vi "Logic.vi"(8 "error in (no error)":errorcluster, 11 "CIFTemplatePlugin in":refnum<class "TemplatePlugin.lvclass">) -> (0 "error out":errorcluster, 3 "CIFTemplatePlugin out":refnum<class "TemplatePlugin.lvclass">)   [LabVIEW 2021, in "TemplatePlugin.lvclass"]
uses:
  TemplatePlugin.lvclass
  D:/dev/CIF-LVCore/src/CIFCore/Class/CIFCorePlugin.lvclass
  TemplatePlugin.lvclass/TemplatePlugin.ctl
  Common/Typedef/Channels.ctl
  CIF-LVCore/src/CIFCore/Class/CIFCorePlugin.lvclass/CIFCorePlugin.ctl
  CIF-LVCore/src/CIFCore/Class/Accessors/Monitor/Write Double 1.vi
  CIF-LVCore/src/CIFCore/Class/Accessors/Monitor/Write U64 1.vi
  CIF-LVCore/src/CIFCore/Class/Accessors/Monitor/Write U64 2.vi
  CIF-LVCore/src/CIFCore/Class/Accessors/Monitor/Write I64 1.vi
  CIF-LVCore/src/CIFCore/Class/Accessors/Monitor/Write I64 2.vi
  <vilib>/CIF Foundation/CIF Channels Core/CIFChannels/CIFChannels.lvclass
  CIF-LVCore/src/CIFCore/Class/CIFCorePlugin.lvclass
  Common/TemplateCommon.lvlib
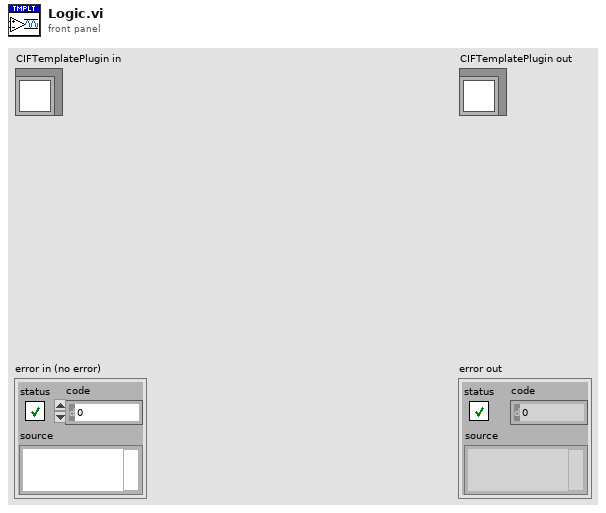
[diagram p1: front panel]
types:
  T1 = typedef "TemplateCommon.lvlib/Channels.ctl" = enum16{"doubleout", "doublein1", "doublein2", "uint_out", "uint_in", "u8array_out", "u8array_in"}
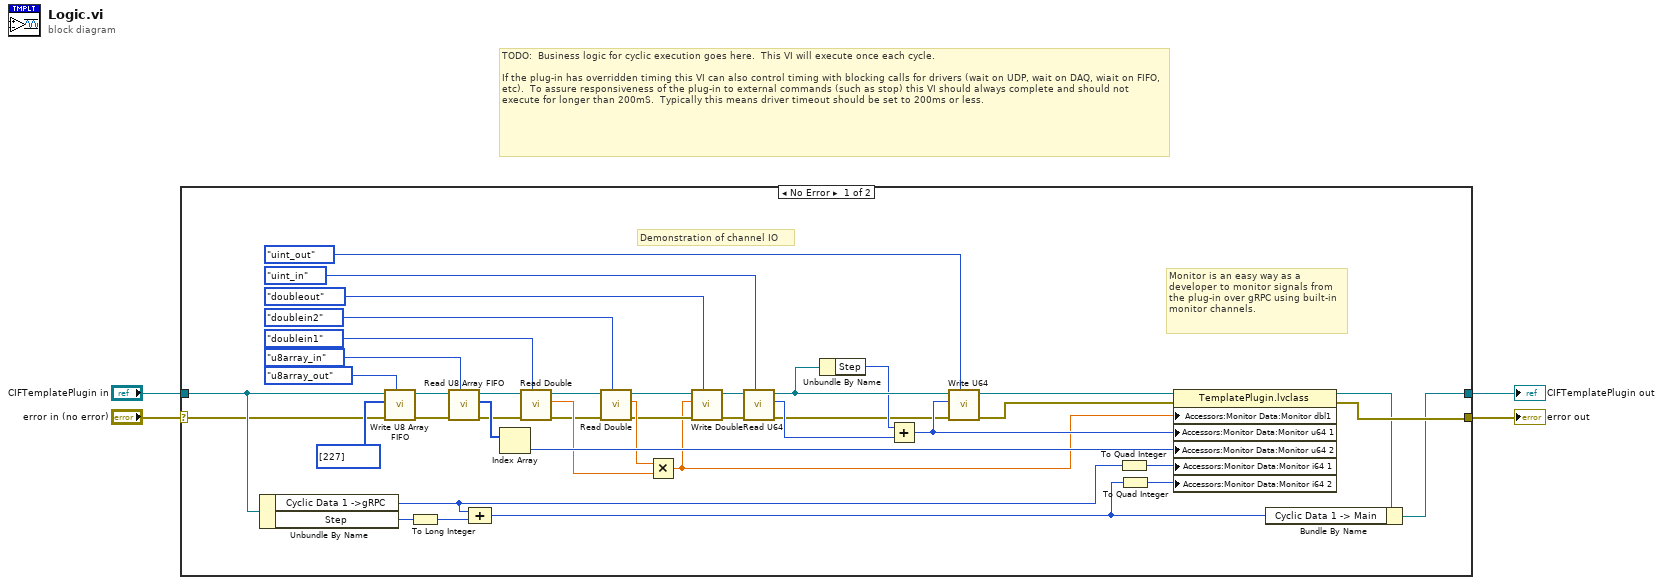
[diagram p0: block diagram]
diagram:
  # "TODO:  Business logic for cyclic execution goes here.  This VI will execute once each cycle.  \n\nIf the plug-in has overridden timing this VI can also control timing with blocking calls for drivers (wait on UDP, wait on DAQ, wiait on FIFO, etc).  To assure responsiveness of the plug-in to external commands (such as stop) this VI should always complete and should not execute for longer than 200mS.  Typically this means driver timeout should be set to 200ms or less."
  n1 = case shown="No Error" "error in (no error)" {
    selector: "error in (no error)" -> [w5 w47]
    tunnel: [w45 w47] -> w2
    tunnel: [w37 w46] -> w1
    tunnel: "CIFTemplatePlugin in" -> [w28 w46]
    frame No Error {
      # "Demonstration of channel IO"
      # "Monitor is an easy way as a developer to monitor signals from the plug-in over gRPC using built-in monitor channels."
      n2 = Unbundle By Name(w28) -> ("Cyclic Data 1 ->gRPC"=w42:i32, "Step"=w35:u64)
      n3 = call "Write U8 Array FIFO.vi"("Channel Index"=Channels."u8array_out" ("Channels"), "error in (no error)"=w5, "Data"=u8[] [227] ("Data in"), "CIFCorePlugin in"=w28) -> ("error out"=w6:errorcluster, "CIFCorePlugin out"=w25:refnum<class "TemplatePlugin.lvclass">)  [unwired: 5 in, 1 out]
      n4 = To Long Integer(number=w35) -> (32bit integer=w43:i32)
      n5 = call "Read U8 Array FIFO.vi"("Channel Index"=Channels."u8array_in" ("Channels"), "error in (no error)"=w6, "CIFCorePlugin in"=w25) -> ("error out"=w7:errorcluster, "Data"=w23:u8[], "CIFCorePlugin out"=w19:refnum<class "TemplatePlugin.lvclass">)  [unwired: 4 in, 2 out]
      n6 = Compound Arithmetic op=ADD(w42, w43) -> (w41:i32)
      n7 = Index Array(array=w23) -> (element=w30:u8)  [unwired: 1 in]
      n8 = call "Read Double.vi"("Channel Index"=Channels."doublein1" ("Channels"), "error in (no error)"=w7, "CIFCorePlugin in"=w19) -> ("error out"=w17:errorcluster, "Data"=w18:dbl, "CIFCorePlugin out"=w16:refnum<class "TemplatePlugin.lvclass">)  [unwired: 6 in]
      n9 = call "Read Double.vi"("Channel Index"=Channels."doublein2" ("Channels"), "error in (no error)"=w17, "CIFCorePlugin in"=w16) -> ("error out"=w14:errorcluster, "Data"=w15:dbl, "CIFCorePlugin out"=w13:refnum<class "TemplatePlugin.lvclass">)  [unwired: 6 in]
      n10 = Multiply(x=w15, y=w18) -> (x*y=w12:dbl)
      n11 = call "Write Double.vi"("Channel Index"=Channels."doubleout" ("Channels"), "error in (no error)"=w14, "Data"=w12, "CIFCorePlugin in"=w13) -> ("error out"=w10:errorcluster, "CIFCorePlugin out"=w11:refnum<class "TemplatePlugin.lvclass">)  [unwired: 6 in]
      n12 = call "Read U64.vi"("Channel Index"=Channels."uint_in" ("Channels"), "error in (no error)"=w10, "CIFCorePlugin in"=w11) -> ("error out"=w8:errorcluster, "Data"=w33:u64, "CIFCorePlugin out"=w34:refnum<class "TemplatePlugin.lvclass">)  [unwired: 6 in]
      n13 = Unbundle By Name(w34) -> ("Step"=w32:u64)
      n14 = Add(x=w32, y=w33) -> (x+y=w31:u64)
      n15 = call "Write U64.vi"("Channel Index"=Channels."uint_out" ("Channels"), "error in (no error)"=w8, "Data"=w31, "CIFCorePlugin in"=w34) -> ("error out"=w9:errorcluster, "CIFCorePlugin out"=w29:refnum<class "TemplatePlugin.lvclass">)  [unwired: 6 in]
      n16 = To Quad Integer(1:w42) -> (0:w40:i64)
      n17 = To Quad Integer(1:w41) -> (0:w39:i64)
      n18 = property class="TemplatePlugin.lvclass"(reference=w29, error in=w9, "Accessors:Monitor Data:Monitor dbl1"=w12, "Accessors:Monitor Data:Monitor u64 1"=w31, "Accessors:Monitor Data:Monitor u64 2"=w30, "Accessors:Monitor Data:Monitor i64 1"=w40, "Accessors:Monitor Data:Monitor i64 2"=w39) -> (reference out=w38:refnum<class "TemplatePlugin.lvclass">, error out=w45:errorcluster)
      n19 = Bundle By Name(cluster=w38, "Cyclic Data 1 -> Main"=w41) -> (w37:refnum<class "TemplatePlugin.lvclass">)
    }
    frame Error {
    }
  }
  "error out" <- w2
  "CIFTemplatePlugin out" <- w1
